vi "Thermal_Camera_Stream.vi"() -> ()   [LabVIEW 2022 SP3]
uses:
  <vilib>/userdefined/High Color/IMAQdx.ctl
  <vilib>/vision/driver/NI_Vision_Acquisition_Software.lvlib
  <resource>/objmgr/imaqdx.rc
panel:
  in  "save":bool
  out "FocusPos":u32
  in  "Scale":u32=13
  in  "Focus >":bool
  in  "Focus <":bool
  in  "Focus":bool
  in  "Numeric":u16
  in  "path":string
  out "error out":errorcluster
  in  "Stop":bool
  in  "Session In":T1="cam4"
  out "Image":T2(plugin-control)
  out "Intensity Graph 2":dbl[][](graph)
  out "Temperature":dbl
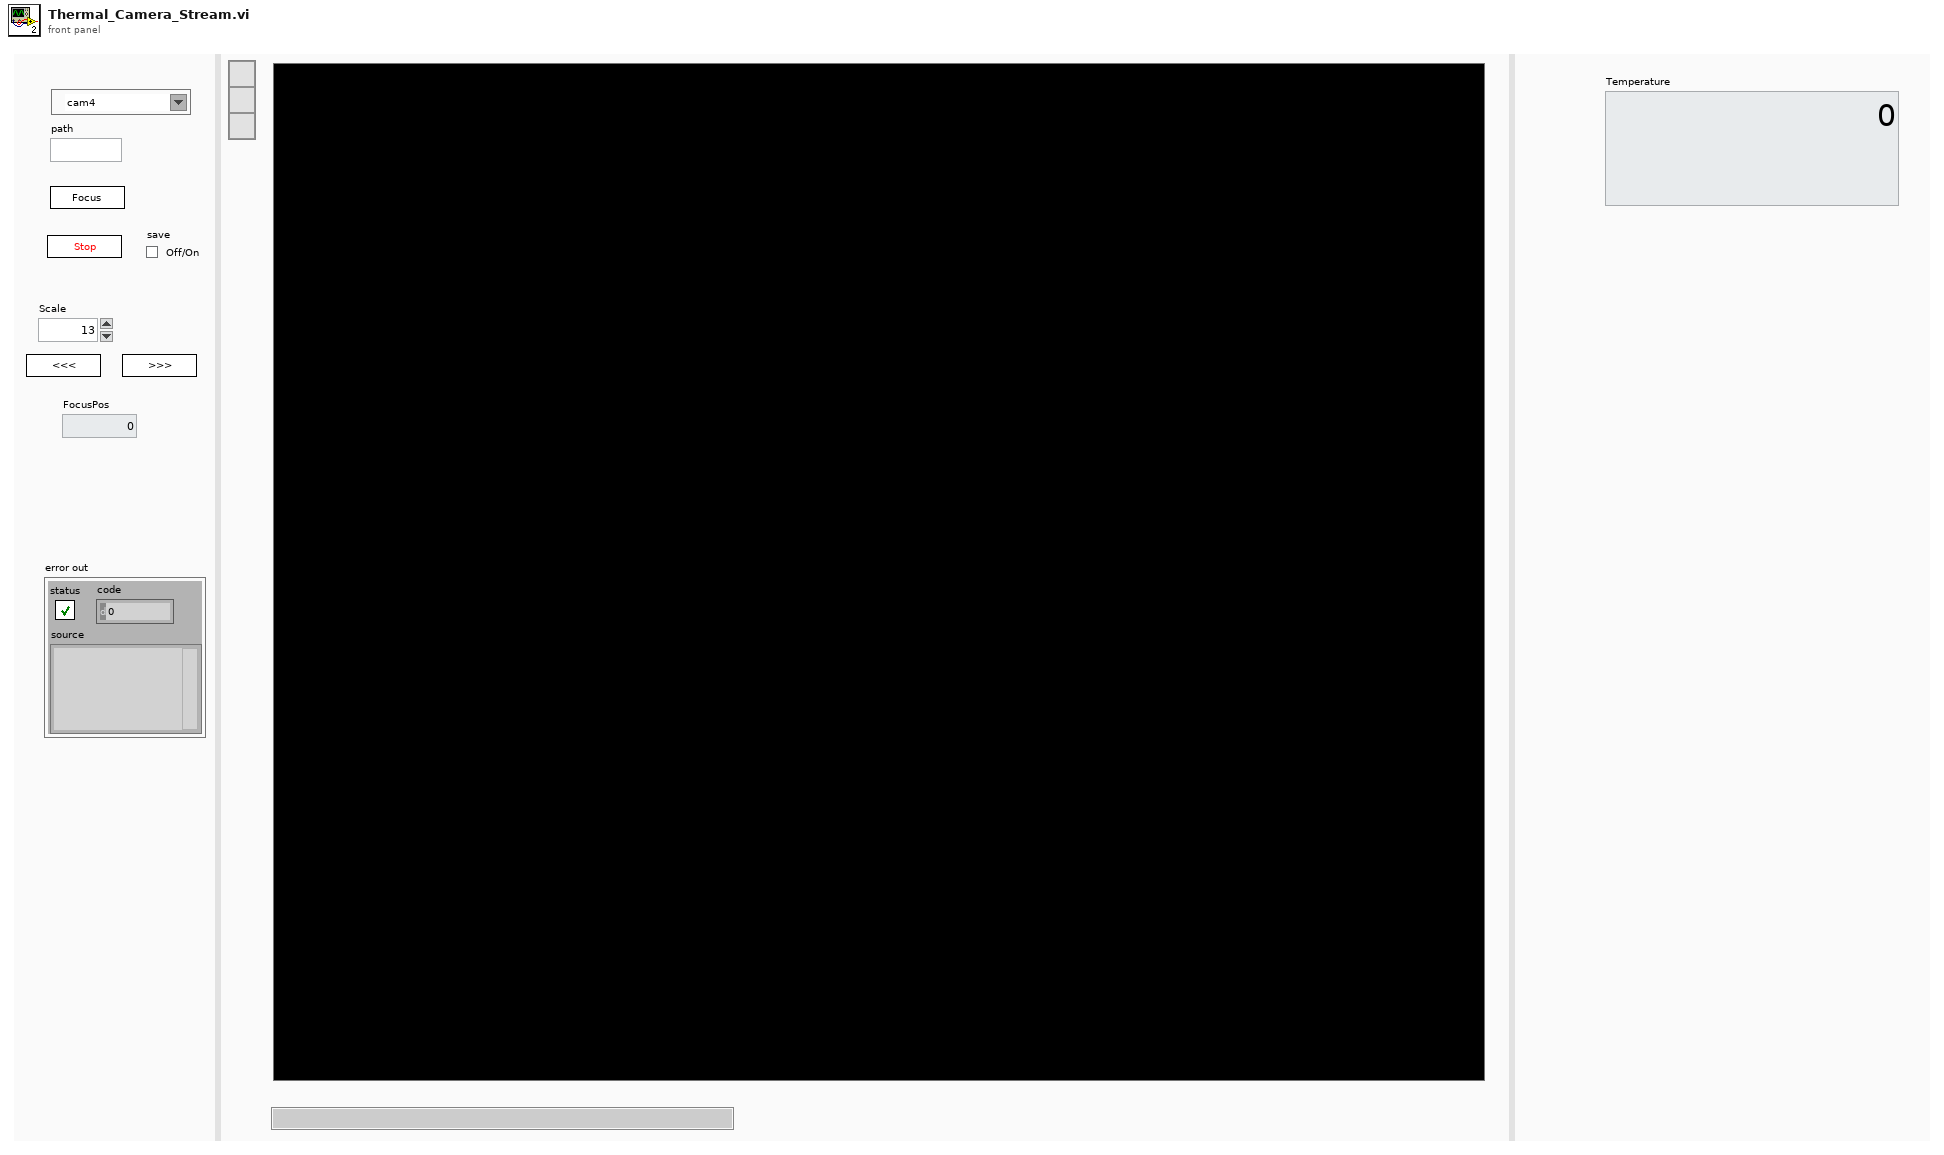
[diagram p1: front panel]
types:
  T1 = typedef "IMAQdx.ctl" = refnum<k21>
  T2 = typedef "IMAQ Image.ctl" = refnum<image>
  T3 = typedef "Image Type" = u32
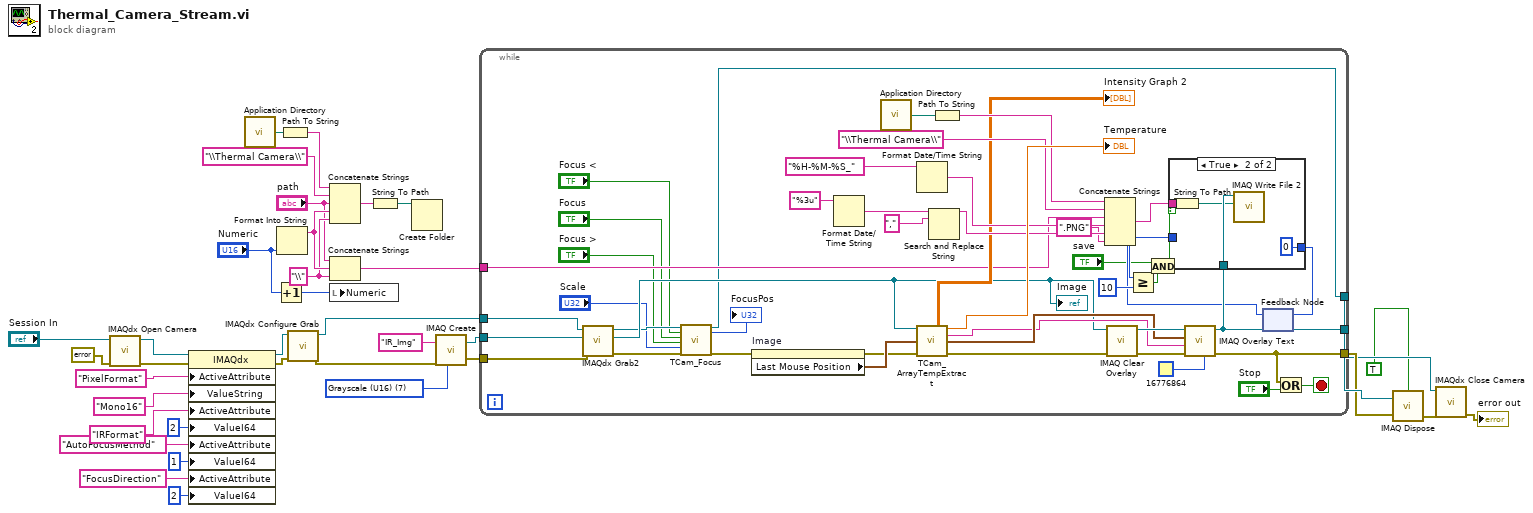
[diagram p0: block diagram]
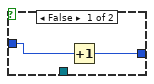
[diagram p2: hidden frame]
diagram:
  w9 = "\\" ("string")
  w21 = T3 7 items=["Grayscale (U8)", "Grayscale (I16)", "Grayscale (SGL)", "Complex (CSG)", "RGB (U32)", "HSL (U32)", "RGB (U64)", "Grayscale (U16)"] ("Image Type")
  n1 = call <vilib>:"IMAQdx Open Camera.vi"("error in"=errorcluster {"status"=FALSE, "code"=0, "source"=""}, "Session In"="Session In") -> ("error out"=w36:errorcluster, "Session Out"=w37:T1)  [unwired: 8 in]
  n2 = property class="IMAQdx"(reference=w37, error in=w36, "ActiveAttribute"="PixelFormat", "ValueString"="Mono16", "ActiveAttribute"="IRFormat", "ValueI64"=i64 2, "ActiveAttribute"="AutoFocusMethod", "ValueI64"=i64 1, "ActiveAttribute"="FocusDirection", "ValueI64"=i64 2) -> (reference out=w2:T1, error out=w1:errorcluster)
  n3 = call <vilib>:"Application Directory.vi"() -> ("Application Directory"=w20:path)
  n4 = Increment(x="Numeric") -> (x+1=w14:u16)
  n5 = Format Into String("Numeric") -> (resulting string=w10:string)  [unwired: 3 in, 1 out]
  n6 = Path To String(path=w20) -> (string=w18:string)
  n7 = call <vilib>:"IMAQdx Configure Grab.vi"("error in"=w1, "Session In"=w2) -> ("error out"=w33:errorcluster, "Session Out"=w34:T1)  [unwired: 8 in]
  n8 = Concatenate Strings(w18, "\\Thermal Camera\\", "path", w10, w9) -> (w17:string)
  n9 = Concatenate Strings("path", w10, w9) -> (w7:string)
  n10 = local write "Numeric"(w14) -> ()
  n11 = String To Path(string=w17) -> (path=w16:path)
  n12 = Create Folder(path (use dialog)=w16) -> ()  [unwired: 2 in, 3 out]
  n13 = call "IMAQ Create"("Image Name"="IR_Img", "Image Type"=w21, "error in (no error)"=w33) -> ("New Image"=w12:T2, "error out"=w11:errorcluster)  [unwired: 2 in]
  n14 = while {
    tunnel: w34 -> [w80]
    tunnel: w11 -> [w79]
    tunnel: [w68] -> w32
    tunnel: [w75] -> w31
    tunnel: [w41] -> w29
    tunnel: w12 -> [w51]
    tunnel: w7 -> [w50]
    stop <- w81 stop-if-true
    n15 = call <vilib>:"IMAQdx Grab2.vi"("error in"=w79, "Image In"=w51, "Session In"=w80) -> ("error out"=w47:errorcluster, "Image Out"=w49:T2, "Session Out"=w48:T1)  [unwired: 5 in, 1 out]
    "Image" <- w49
    n16 = call "TCam_Focus.vi"("Session in"=w48, "Focus <"="Focus <", "Autofocus"="Focus", "Focus >"="Focus >", "Scale"="Scale", "error in (no error)"=w47) -> ("Session Out"=w41:T1, "FocusPos"=→"FocusPos":u32, "error out"=w42:errorcluster)  [unwired: 11 in]
    n17 = property on="Image" class="ImageControl"(error in=w42) -> (error out=w71:errorcluster, "Last Mouse Position"=w72:cluster{"X":i32, "Y":i32})  [unwired: 1 in, 1 out]
    n18 = Format Date/Time String(time format string (%c)="%3u") -> (date/time string=w66:string)  [unwired: 2 in]
    n19 = call <vilib>:"Application Directory.vi"() -> ("Application Directory"=w61:path)
    n20 = Format Date/Time String(time format string (%c)="%H-%M-%S_") -> (date/time string=w65:string)  [unwired: 2 in]
    n21 = call "TCam_ArrayTempExtract.vi"("img in"=w49, "Mouse pos"=w72, "error in (no error)"=w71) -> ("Intensity Graph 4"=→"Intensity Graph 2":dbl[][], "temp"=→"Temperature":dbl, "temp str"=w69:string, "Mouse pos dup"=w70:cluster{"X":i32, "Y":i32}, "error out"=w73:errorcluster)  [unwired: 8 in]
    n22 = Search and Replace String(input string=w66, search string=",") -> (result string=w67:string)  [unwired: 6 in, 3 out]
    n23 = Path To String(path=w61) -> (string=w59:string)
    n24 = Concatenate Strings(w59, "\\Thermal Camera\\", w50, w65, w67, ".PNG" ("string")) -> (w57:string)
    n25 = call "IMAQ Clear Overlay"("error in (no error)"=w73, "Image"=w49) -> ("error out"=w76:errorcluster, "Image Out"=w77:T2)  [unwired: 8 in]
    n26 = call "IMAQ Overlay Text"("BG Color (Transparent)"=u32 16776864, "error in (no error)"=w76, "String"=w69, "Origin"=w70, "Image"=w77) -> ("error out"=w75:errorcluster, "Image Out"=w68:T2)  [unwired: 5 in]
    n27 = feedback #1() -> (w53:u16)  [unwired: 1 in]
    n28 = Greater Or Equal?(x=w53, y=u16 10) -> (x >= y?=w56:bool)
    n29 = And(x="save", y=w56) -> (x .and. y?=w39:bool)
    n30 = case shown="True" w39 {
      tunnel: w68 -> [_ w88]
      tunnel: w57 -> [_ w87]
      tunnel: [w83 u16 0 ("y")] -> w54
      tunnel: w53 -> [w84 _]
      frame False {
        n31 = Increment(x=w84) -> (x+1=w83:u16)
      }
      frame True {
        n32 = String To Path(string=w87) -> (path=w86:path)
        n33 = call-poly "IMAQ Write File 2"("File Path"=w86, "Image"=w88) -> ()  [unwired: 8 in, 2 out]
      }
    }
    n34 = feedback-in #1(w54) -> ()
    n35 = Or(x=w75, y="Stop") -> (x .or. y?=w81:bool)
  }
  n36 = call "IMAQ Dispose"("All Images? (No)"=TRUE, "Image"=w32, "error in (no error)"=w31) -> ("error out"=w30:errorcluster)  [unwired: 3 in]
  n37 = call <vilib>:"IMAQdx Close Camera.vi"("error in"=w30, "Session In"=w29) -> ("error out"=→"error out":errorcluster)  [unwired: 9 in]
